vi "LockinDSP.TestLauncher.vi"() -> ()   [LabVIEW 2016, in "LockinDSP.lvclass"]
uses:
  LockinDSP.lvclass
  <vilib>/JKI/JKI SMO/SMO/Typedefs/SMOState --Enum.ctl
  C:/Program Files (x86)/National Instruments/LabVIEW 2016/vi.lib/JKI/JKI SMO/SMO/SMO.lvclass
  <vilib>/JKI/JKI SMO/SMO/SMO.lvclass
panel:
  out "SMO State":T1
  out "error out":errorcluster
  in  "Stop":bool
  # "Basic SMO Test Launcher"
  # "For instructions on how to use the JKI State Machine Objects, examples and video tutorials, visit:\nhttp://jki.net/state-machine-objects/\n\nJKI State Machine Objects™\nhttp://jki.net/state-machine-objects/\nCopyright (C) 2005-2015, JKI <info@jki.net>\nALL RIGHTS RESERVED"
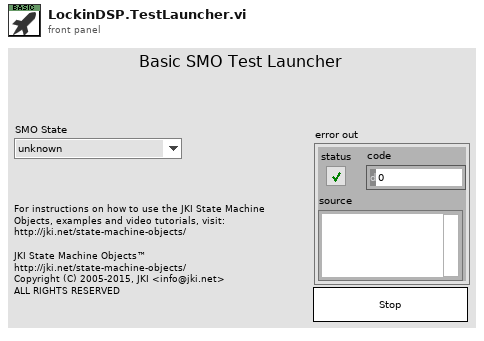
[diagram p1: front panel]
types:
  T1 = typedef "SMO.lvclass/SMOState --Enum.ctl" = enum16{"unknown", "Created", "Started", "Stopped"}
  T2 = typedef "SMO.lvclass/Public Events.ctl" = cluster{"Error":refnum<user-event>, "State":refnum<user-event>, "Reserve State":refnum<user-event>}
  T3 = cluster{"Event Registration Refnum":refnum<event-registration>}
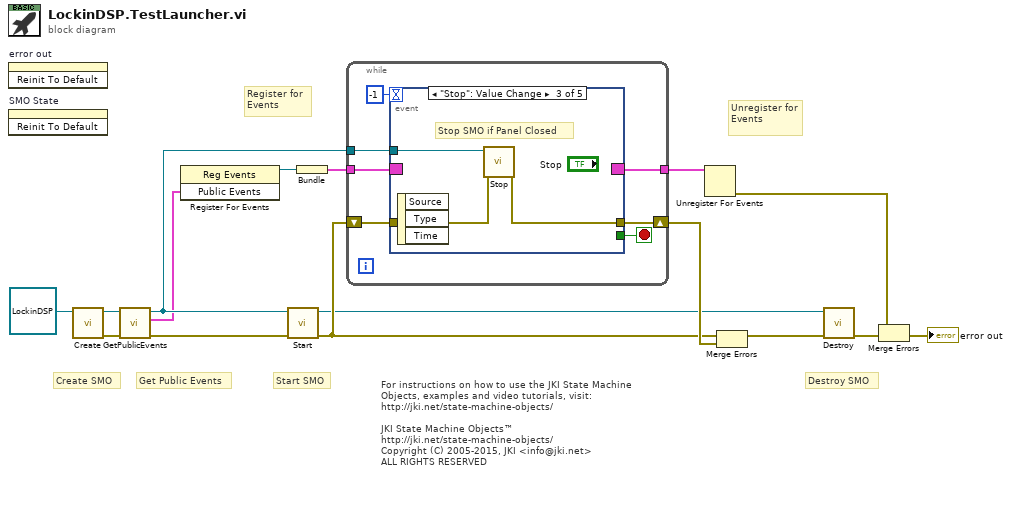
[diagram p0: block diagram]
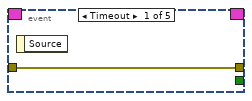
[diagram p2: hidden frame]
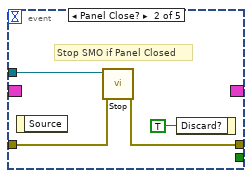
[diagram p3: hidden frame]
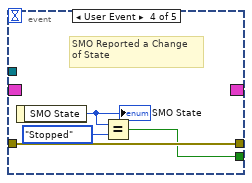
[diagram p4: hidden frame]
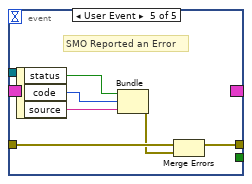
[diagram p5: hidden frame]
diagram:
  # "For instructions on how to use the JKI State Machine Objects, examples and video tutorials, visit:\nhttp://jki.net/state-machine-objects/\n\nJKI State Machine Objects™\nhttp://jki.net/state-machine-objects/\nCopyright (C) 2005-2015, JKI <info@jki.net>\nALL RIGHTS RESERVED"
  # "Get Public Events"
  # "Start SMO"
  # "Destroy SMO"
  # "Create SMO"
  # "Unregister for Events"
  # "Register for Events"
  n1 = invoke on="error out" class="Clust (strict)" method="Reinit To Default"() -> ()  [unwired: 3 in, 3 out]
  n2 = invoke on="SMO State" class="Enum (strict)" method="Reinit To Default"() -> ()  [unwired: 3 in, 3 out]
  n3 = call <vilib>:"Create.vi"("SMO"=refnum<class "LockinDSP.lvclass"> refnum ("SMO.Template.lvclass")) -> ("error out"=w5:errorcluster, "SMO out"=w6:refnum<class "LockinDSP.lvclass">)  [unwired: 8 in, 1 out]
  n4 = call <vilib>:"GetPublicEvents.vi"("error in (no error)"=w5, "SMO"=w6) -> ("error out"=w4:errorcluster, "Public Events"=w2:T2, "SMO out"=w3:refnum<class "LockinDSP.lvclass">)  [unwired: 7 in]
  n5 = register-events(w2) -> (reference out=w1:refnum<event-registration>)  [unwired: 2 in, 1 out]
  n6 = call <vilib>:"Start.vi"("error in (no error)"=w4, "SMO"=w3) -> ("error out"=w9:errorcluster, "SMO out"=w7:refnum<class "LockinDSP.lvclass">)  [unwired: 8 in]
  n7 = Bundle("Event Registration Refnum"=w1) -> (w15:T3)  [unwired: 1 in]
  n8 = while {
    shift-right: [w22] -> w14
    shift-left: w9 -> [w21]
    tunnel: w15 -> [w20]
    tunnel: [w19] -> w16
    tunnel: w3 -> [w18]
    stop <- w23 stop-if-true
    n9 = event shown="[2] \"Stop\": Value Change" {
      selector: w20 -> [_ _ _ _ _]
      dyn-events: [_ _ _ _ _] -> w19
      timeout: -1 -> [_ _ _ _ _]
      tunnel: [_ _ _ w32 _] -> w23
      tunnel: w18 -> [_ w28 w31 _ _]
      tunnel: [w24 w27 w30 w35 w39] -> w22
      tunnel: w21 -> [w24 w26 w29 w35 w37]
      event Timeout {
        n10 = event-data() -> ()  [unwired: 1 in, 1 out]
      }
      event Panel Close? {
        # "Stop SMO if Panel Closed"
        n11 = event-data() -> ()  [unwired: 1 in, 1 out]
        n12 = call <vilib>:"Stop.vi"("error in (no error)"=w26, "SMO"=w28) -> ("error out"=w27:errorcluster)  [unwired: 8 in, 1 out]
        n13 = event-data("Discard?"=TRUE ("OK")) -> ()  [unwired: 1 in, 1 out]
      }
      event "Stop": Value Change {
        # "Stop SMO if Panel Closed"
        n14 = event-data() -> ()  [unwired: 1 in, 3 out]
        n15 = call <vilib>:"Stop.vi"("error in (no error)"=w29, "SMO"=w31) -> ("error out"=w30:errorcluster)  [unwired: 8 in, 1 out]
      }
      event User Event {
        # "SMO Reported a Change\nof State"
        n16 = event-data() -> ("SMO State"=w34:T1)  [unwired: 1 in]
        "SMO State" <- w34
        n17 = Equal?(x=w34, y=SMOState_--Enum."Stopped") -> (x = y?=w32:bool)
      }
      event User Event {
        # "SMO Reported an Error"
        n18 = event-data() -> ("status"=w38:bool, "code"=w41:i32, "source"=w40:string)  [unwired: 1 in]
        n19 = Bundle("status"=w38, "code"=w41, "source"=w40) -> (w36:errorcluster)  [unwired: 1 in]
        n20 = Merge Errors(w37, w36) -> (w39:errorcluster)
      }
    }
  }
  n21 = Unregister For Events(event registration refnum=w16) -> (error out=w13:errorcluster)  [unwired: 1 in]
  n22 = Merge Errors(w9, w14) -> (w8:errorcluster)
  n23 = call <vilib>:"Destroy.vi"("error in (no error)"=w8, "SMO"=w7) -> ("error out"=w11:errorcluster)  [unwired: 9 in]
  n24 = Merge Errors(w13, w11) -> (→"error out":errorcluster)
